vi "arrayeverage.vi"(9 "divider":dbl, 10 "in":dbl[](array[numeric])) -> (2 "out":dbl[](array[numeric]))   [LabVIEW 2012]
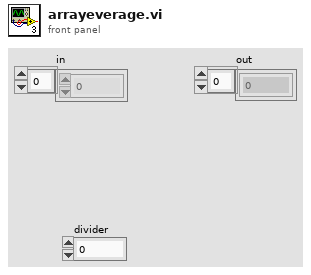
[diagram p1: front panel]
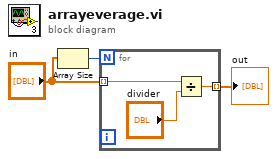
[diagram p0: block diagram]
diagram:
  n1 = Array Size(array="in") -> (size(s)=w3:i32)
  n2 = for {
    N: w3 -> [_]
    tunnel: "in" -> [w5] mode=indexing
    tunnel: [w4] -> w1 mode=indexing
    n3 = Divide(x=w5, y="divider") -> (x/y=w4:dbl)
  }
  "out" <- w1
